vi "p1.vi"() -> ()   [LabVIEW 2023, in "d23.lvlib"]
uses:
  d23.lvlib
  <vilib>/Utility/miscctls.llb/LVMapReplaceAction.ctl
  AOC/AOC.lvlib
panel:
  out "Map":T1(c390)
  in  "Example":string="#.#####################\n#.......#########...###\n#######.#########.#.###\n###.....#.>.>.###.#.###\n###v#####.#v#.###.#.###\n###.>...#.#.#.....#...#\n###v###.#.#.#########.#\n###...#.#.#.......#...#\n#####.#.#.#######.#.###\n#.....#.#.#.......#...#\n#.#####.#.#.#########v#\n#.#...#...#...###...>.#\n#.#.#v#######v###.###v#\n#...#.>.#...>.>.#.###.#\n#####v#.#.###v#.#.###.#\n#.....#...#...#.#.#...#\n#.#########.###.#.#.###\n#...###...#...#...#.###\n###.###.#.###v#####v###\n#...#...#.#.>.>.#.>.###\n#.###.###.#.###.#.#v###\n#.....###...###...#...#\n#####################.#"
  in  "Example":bool=TRUE
  out "Answer":u64
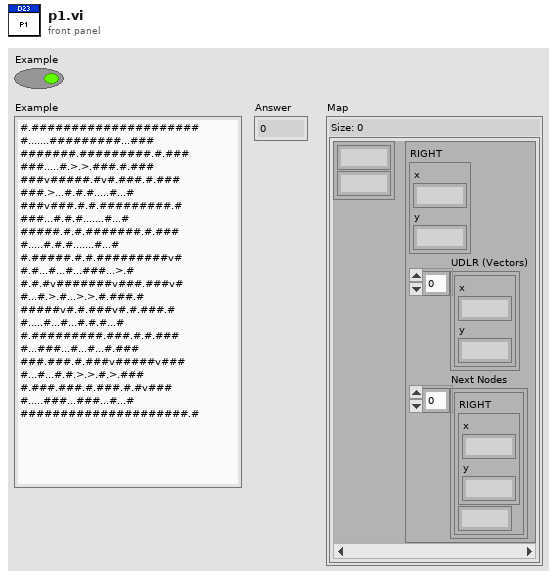
[diagram p1: front panel]
types:
  T1 = map{cluster{i32, i32}, cluster{"RIGHT":cluster{"x":i16, "y":i16}, "UDLR (Vectors)":cluster{"x":i16, "y":i16}[], "Next Nodes":cluster{"RIGHT":cluster{"x":i16, "y":i16}, u64}[]}}
  T2 = cluster{"Location":cluster{i32, i32}, "Previous Nodes":cluster{i32, i32}[], "Node Distance":u64, "Direction":cluster{"x":i16, "y":i16}}
  T3 = cluster{"RIGHT":cluster{"x":i16, "y":i16}, u64}[]
  T4 = cluster{"RIGHT":cluster{"x":i16, "y":i16}, "UDLR (Vectors)":cluster{"x":i16, "y":i16}[], "Next Nodes":cluster{"RIGHT":cluster{"x":i16, "y":i16}, u64}[]}
  T5 = typedef "LVMapReplaceAction.ctl" = enum32{"Modify Entry only if found", "Add or Modify Entry", "Delete Entry"}
  T6 = cluster{"Location":cluster{i32, i32}, "Node Distance":u64}
  T7 = cluster{"Location":cluster{"x":i32, "y":i32}, "Node Distance":u64}[]
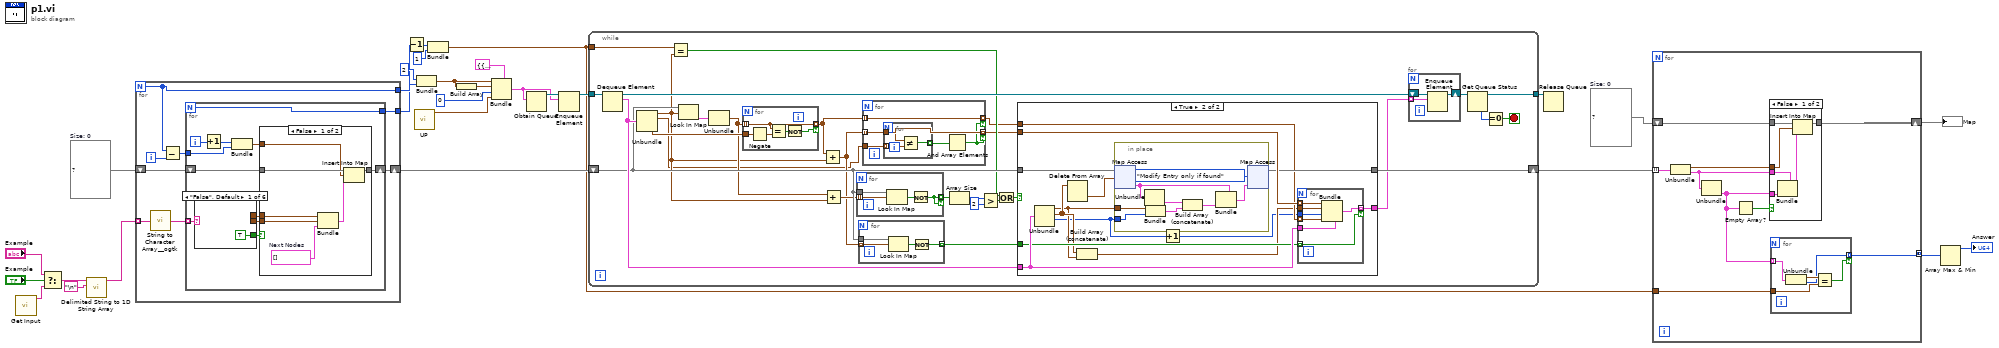
[diagram p0: block diagram]
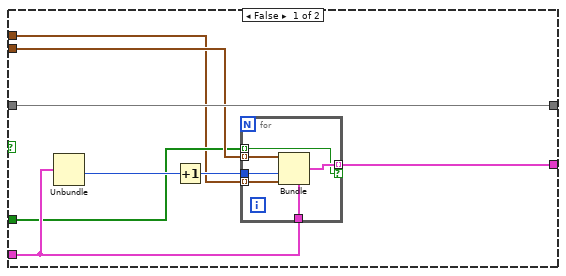
[diagram p2: hidden frame]
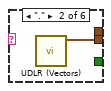
[diagram p3: hidden frame]
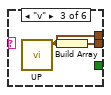
[diagram p4: hidden frame]
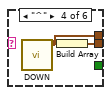
[diagram p5: hidden frame]
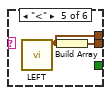
[diagram p6: hidden frame]
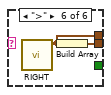
[diagram p7: hidden frame]
diagram:
  w10 = T1 {}  # Size: 0
  w22 = T1 {}  # Size: 0
  n1 = call "Get Input.vi"() -> ("Input"=w28:string)  [unwired: 11 in]
  n2 = Select(t="Example", s="Example", f=w28) -> (s? t:f=w27:string)
  n3 = call <vilib>:"Delimited String to 1D String Array.vi"("delimiter"="\n", "delimited string"=w27) -> ("string array"=w23:string[])  [unwired: 9 in]
  n4 = for {
    N -> [w30]
    tunnel: w23 -> [w36] mode=indexing
    shift-right: [w31] -> w21
    shift-left: w22 -> [w32]
    tunnel: [w30] -> w16
    tunnel: [w29] -> w8
    i -> [w34]
    n5 = call <userlib>:"String to Character Array__ogtk.vi"("Input String"=w36) -> ("Character Array"=w35:string[])
    n6 = Subtract(x=w30, y=w34) -> (x-y=w33:i32)
    n7 = for {
      N -> [w37]
      tunnel: w35 -> [w39] mode=indexing
      tunnel: w33 -> [w45]
      shift-right: [w44] -> w31
      shift-left: w32 -> [w43]
      tunnel: [w37] -> w29
      i -> [w47]
      n8 = case shown="\"False\", Default" w39 {
        tunnel: [_ w49 w51 w53 w55 w57] -> w41
        tunnel: [TRUE _ _ _ _ _] -> w40
        tunnel: [_ _ w50 w52 w54 w56] -> w38
        frame "False", Default {
        }
        frame "." {
          n9 = call "UDLR (Vectors).vi"() -> ("UDLR (Vectors)"=w49:cluster{"x":i16, "y":i16}[])  [unwired: 11 in]
        }
        frame "v" {
          n10 = call "UP.vi"() -> ("UP"=w50:cluster{"x":i16, "y":i16})  [unwired: 11 in]
          n11 = Build Array(w50) -> (w51:cluster{"x":i16, "y":i16}[])
        }
        frame "^" {
          n12 = call "DOWN.vi"() -> ("DOWN"=w52:cluster{"x":i16, "y":i16})  [unwired: 11 in]
          n13 = Build Array(w52) -> (w53:cluster{"x":i16, "y":i16}[])
        }
        frame "<" {
          n14 = call "LEFT.vi"() -> ("LEFT"=w54:cluster{"x":i16, "y":i16})  [unwired: 11 in]
          n15 = Build Array(w54) -> (w55:cluster{"x":i16, "y":i16}[])
        }
        frame ">" {
          n16 = call "RIGHT.vi"() -> ("RIGHT"=w56:cluster{"x":i16, "y":i16})  [unwired: 11 in]
          n17 = Build Array(w56) -> (w57:cluster{"x":i16, "y":i16}[])
        }
      }
      n18 = Increment(x=w47) -> (x+1=w46:i32)
      n19 = Bundle(w46, w45) -> (w42:cluster{i32, i32})  [unwired: 1 in]
      n20 = case shown="False" w40 {
        tunnel: [w64 w65] -> w44
        tunnel: w43 -> [w63 w65]
        tunnel: w42 -> [w62 _]
        tunnel: w41 -> [w61 _]
        tunnel: w38 -> [w58 _]
        frame False {
          w59 = T3 []  # Next Nodes
          n21 = Bundle("RIGHT"=w58, "UDLR (Vectors)"=w61, "Next Nodes"=w59) -> (w60:T4)  [unwired: 1 in]
          n22 = Insert Into Map(map in=w63, key=w62, value=w60) -> (map out=w64:T1)  [unwired: 2 out]
        }
        frame True {
        }
      }
    }
  }
  n23 = Decrement(x=w8) -> (x-1=w6:i32)
  n24 = call "UP.vi"() -> ("UP"=w11:cluster{"x":i16, "y":i16})  [unwired: 11 in]
  n25 = Bundle(2, w16) -> (w15:cluster{i32, i32})  [unwired: 1 in]
  n26 = Bundle(w6, 1) -> (w3:cluster{i32, i32})  [unwired: 1 in]
  n27 = Build Array(w15) -> (w4:cluster{i32, i32}[])
  n28 = Bundle(cluster=T2 {"Location"={0, 0}, "Previous Nodes"=[], "Node Distance"=0, "Direction"={"x"=0, "y"=0}}, "Location"=w15, "Previous Nodes"=w4, "Node Distance"=u64 0, "Direction"=w11) -> (w14:T2)
  n29 = Obtain Queue(element data type=w14) -> (queue out=w19:refnum<queue>)  [unwired: 4 in, 2 out]
  n30 = Enqueue Element(queue=w19, element=w14) -> (queue out=w18:refnum<queue>)  [unwired: 2 in, 2 out]
  n31 = while {
    shift-right: [w86] -> w12
    shift-left: w21 -> [w80]
    tunnel: w18 -> [w93]
    tunnel: [w88] -> w17
    tunnel: w3 -> [w74]
    stop <- w89 stop-if-true
    n32 = Dequeue Element(queue=w93) -> (queue out=w92:refnum<queue>, element=w85:T2)  [unwired: 2 in, 2 out]
    n33 = Unbundle(w85) -> ("Location"=w73:cluster{i32, i32}, "Previous Nodes"=w68:cluster{i32, i32}[], "Direction"=w82:cluster{"x":i16, "y":i16})  [unwired: 1 out]
    n34 = Equal?(x=w74, y=w73) -> (x = y?=w71:bool)
    n35 = Look In Map(map=w80, key=w73) -> (value=w87:T4)  [unwired: 1 in, 1 out]
    n36 = Unbundle(w87) -> ("UDLR (Vectors)"=w79:cluster{"x":i16, "y":i16}[])  [unwired: 2 out]
    n37 = for {
      tunnel: w82 -> [w114]
      tunnel: w79 -> [w112] mode=indexing
      tunnel: [w112] -> w70 mode=indexing if=w110
      n38 = Negate(x=w114) -> (-x=w111:cluster{"x":i16, "y":i16})
      n39 = Equal?(x=w112, y=w111) -> (x = y?=w113:bool)
      n40 = Not(x=w113) -> (.not. x?=w110:bool)
    }
    n41 = Add(x=w70, y=w73) -> (x+y=w69:cluster{i32, i32}[])
    n42 = Add(x=w79, y=w73) -> (x+y=w78:cluster{i32, i32}[])
    n43 = for {
      tunnel: w78 -> [w104] mode=indexing
      tunnel: [w102] -> w81 mode=indexing if=w102
      tunnel: w80 -> [w103]
      n44 = Look In Map(map=w103, key=w104) -> (key not found?=w105:bool)  [unwired: 1 in, 1 out]
      n45 = Not(x=w105) -> (.not. x?=w102:bool)
    }
    n46 = for {
      tunnel: w69 -> [w107] mode=indexing
      tunnel: [w109] -> w83 mode=indexing
      tunnel: w80 -> [w106]
      n47 = Look In Map(map=w106, key=w107) -> (key not found?=w108:bool)  [unwired: 1 in, 1 out]
      n48 = Not(x=w108) -> (.not. x?=w109:bool)
    }
    n49 = for {
      tunnel: w70 -> [w97] mode=indexing
      tunnel: w69 -> [w96] mode=indexing
      tunnel: w68 -> [w98]
      tunnel: [w97] -> w67 mode=indexing if=w94
      tunnel: [w96] -> w66 mode=indexing if=w94
      n50 = for {
        tunnel: w98 -> [w101] mode=indexing
        tunnel: w96 -> [w100]
        tunnel: [w99] -> w95 mode=indexing
        n51 = Not Equal?(x=w100, y=w101) -> (x != y?=w99:bool)
      }
      n52 = And Array Elements(Boolean array=w95) -> (logical AND=w94:bool)
    }
    n53 = Array Size(array=w81) -> (size(s)=w77:i32)
    n54 = Greater?(x=w77, y=2) -> (0:w76:bool)
    n55 = Or(x=w71, y=w76) -> (x .or. y?=w72:bool)
    n56 = case shown="True" w72 {
      tunnel: w80 -> [w122 w141]
      tunnel: w66 -> [w120 w138]
      tunnel: [w122 w136] -> w86
      tunnel: [w119 w140] -> w84
      tunnel: w85 -> [w118 w139]
      tunnel: w83 -> [w116 w137]
      tunnel: w67 -> [w115 w135]
      frame False {
        n57 = Unbundle(w118) -> ("Node Distance"=w117:u64)  [unwired: 3 out]
        n58 = Increment(x=w117) -> (x+1=w121:u64)
        n59 = for {
          tunnel: w121 -> [w128]
          tunnel: w120 -> [w127] mode=indexing
          tunnel: [w126] -> w119 mode=indexing if=w124
          tunnel: w118 -> [w125]
          tunnel: w116 -> [w124] mode=indexing
          tunnel: w115 -> [w123] mode=indexing
          n60 = Bundle(cluster=w125, "Location"=w127, "Node Distance"=w128, "Direction"=w123) -> (w126:T2)  [unwired: 1 in]
        }
      }
      frame True {
        n61 = Unbundle(w139) -> ("Location"=w132:cluster{i32, i32}, "Previous Nodes"=w133:cluster{i32, i32}[], "Node Distance"=w130:u64)  [unwired: 1 out]
        n62 = Delete From Array(array=w133) -> (deleted portion=w134:cluster{i32, i32})  [unwired: 2 in, 1 out]
        n63 = Build Array (concatenate)(w133, w132) -> (w131:cluster{i32, i32}[])
        n64 = in-place {
          in-place-border: w132 -> [w150]
          in-place-border: w130 -> [w149]
          n65 = in-place-map #1(w141, w134) -> (w154:T4)  [unwired: 1 in, 1 out]
          n66 = Unbundle(w154) -> ("Next Nodes"=w156:T3)  [unwired: 2 out]
          n67 = Bundle("Location"=w150, "Node Distance"=w149) -> (w155:T6)  [unwired: 1 in]
          n68 = Build Array (concatenate)(w156, w155) -> (w153:T7)
          n69 = Bundle(cluster=w154, "Next Nodes"=w153) -> (w152:T4)  [unwired: 2 in]
          n70 = in-place-map #1(w152, LVMapReplaceAction."Modify Entry only if found" ("action")) -> (w136:T1)  [unwired: 2 out]
        }
        n71 = Increment(x=w130) -> (x+1=w129:u64)
        n72 = for {
          tunnel: w139 -> [w148]
          tunnel: w129 -> [w147]
          tunnel: w138 -> [w146] mode=indexing
          tunnel: [w145] -> w140 mode=indexing if=w144
          tunnel: w137 -> [w144] mode=indexing
          tunnel: w131 -> [w143]
          tunnel: w135 -> [w142] mode=indexing
          n73 = Bundle(cluster=w148, "Location"=w146, "Previous Nodes"=w143, "Node Distance"=w147, "Direction"=w142) -> (w145:T2)
        }
      }
    }
    n74 = for {
      shift-right: [w158] -> w91
      shift-left: w92 -> [w159]
      tunnel: w84 -> [w157] mode=indexing
      n75 = Enqueue Element(queue=w159, element=w157) -> (queue out=w158:refnum<queue>)  [unwired: 2 in, 2 out]
    }
    n76 = Get Queue Status(queue=w91) -> (queue out=w88:refnum<queue>, # elements in queue=w90:i32)  [unwired: 2 in, 6 out]
    n77 = Equal To 0?(x=w90) -> (x = 0?=w89:bool)
  }
  n78 = Release Queue(queue=w17) -> ()  [unwired: 2 in, 3 out]
  n79 = for {
    tunnel: w12 -> [w168] mode=indexing
    shift-right: [w167] -> w9
    shift-left: w10 -> [w166]
    tunnel: w3 -> [w161]
    tunnel: [w160] -> w2 mode=concatenating
    n80 = Unbundle(w168) -> ("output cluster"=w164:cluster{i32, i32}, "output cluster"=w163:T4)
    n81 = Unbundle(w163) -> ("Next Nodes"=w162:T3)  [unwired: 2 out]
    n82 = Empty Array?(array=w162) -> (empty?=w165:bool)
    n83 = case shown="False" w165 {
      tunnel: [w179 w180] -> w167
      tunnel: w166 -> [w178 w180]
      tunnel: w164 -> [w177 _]
      tunnel: w163 -> [w176 _]
      tunnel: w162 -> [w174 _]
      frame False {
        n84 = Bundle(cluster=w176, "Next Nodes"=w174) -> (w175:T4)  [unwired: 2 in]
        n85 = Insert Into Map(map in=w178, key=w177, value=w175) -> (map out=w179:T1)  [unwired: 2 out]
      }
      frame True {
      }
    }
    n86 = for {
      tunnel: w162 -> [w173] mode=indexing
      tunnel: w161 -> [w171]
      tunnel: [w170] -> w160 mode=indexing if=w169
      n87 = Unbundle(w173) -> ("RIGHT"=w172:cluster{"x":i16, "y":i16}, w170:u64)
      n88 = Equal?(x=w172, y=w171) -> (x = y?=w169:bool)
    }
  }
  "Map" <- w9
  n89 = Array Max & Min(array=w2) -> (max value=→"Answer":u64)  [unwired: 3 out]
